vi "File Paths.vi"() -> (0 "SO45 Settings path":path, 1 "SO55 Settings path":path)   [LabVIEW 2013]
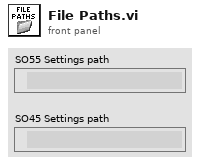
[diagram p1: front panel]
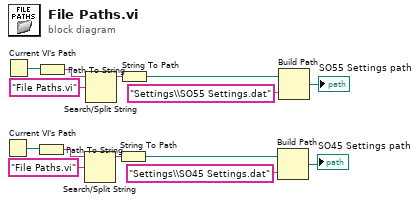
[diagram p0: block diagram]
diagram:
  n1 = Current VI's Path() -> (path=w7:path)
  n2 = Current VI's Path() -> (path=w9:path)
  n3 = Path To String(path=w7) -> (string=w3:string)
  n4 = Path To String(path=w9) -> (string=w13:string)
  n5 = Search/Split String(string=w3, search string/char (-)="File Paths.vi" ("substring (\"\")")) -> (substring before match=w4:string)  [unwired: 1 in, 2 out]
  n6 = Search/Split String(string=w13, search string/char (-)="File Paths.vi" ("substring (\"\")")) -> (substring before match=w12:string)  [unwired: 1 in, 2 out]
  n7 = String To Path(string=w4) -> (path=w5:path)
  n8 = String To Path(string=w12) -> (path=w11:path)
  n9 = Build Path(base path=w5, name or relative path="Settings\\SO45 Settings.dat") -> (appended path=→"SO45 Settings path":path)
  n10 = Build Path(base path=w11, name or relative path="Settings\\SO55 Settings.dat") -> (appended path=→"SO55 Settings path":path)
